vi "Store Panel by Section.vi"(8 "error in (no error)":errorcluster, 9 "Show Status? (T)":bool=TRUE, 10 "VI reference":refnum<vi>, 11 "Path (dialog)":path=path "C:/ProgramData/EPL/CFTS Defaults.ini") -> (0 "Error Out":errorcluster)   [LabVIEW 2020]
doc: "Store the values in the controls of a front panel in a file.\n\nFreeware from Moore Good Ideas, www.mooregoodideas.com. Do not remove this line.\ndavid@mooregoodideas.com"
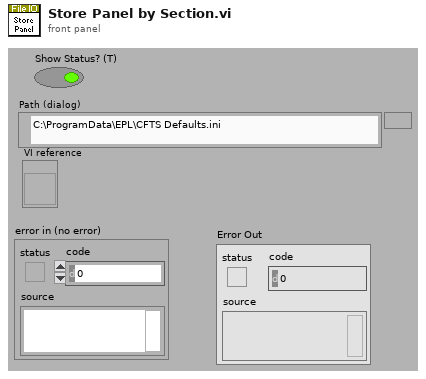
[diagram p1: front panel]
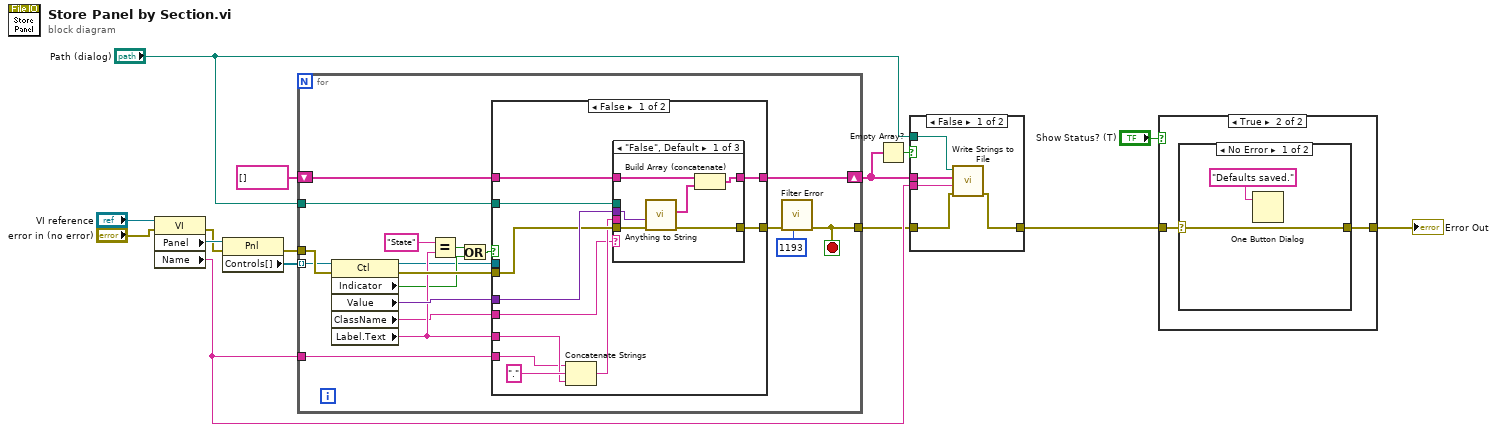
[diagram p0: block diagram]
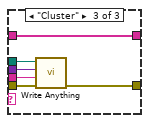
[diagram p4: hidden frame]
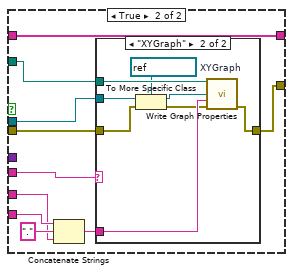
[diagram p5: hidden frame]
diagram:
  n1 = property class="VI"(reference="VI reference", error in="error in (no error)") -> (error out=w10:errorcluster, "Panel"=w11:refnum<vi>, "Name"=w4:string)  [unwired: 1 out]
  n2 = property class="Pnl"(reference=w11, error in=w10) -> (error out=w8:errorcluster, "Controls[]"=w9:refnum<vi>[])  [unwired: 1 out]
  n3 = for {
    tunnel: w9 -> [w27] mode=indexing
    tunnel: w8 -> [w33]
    tunnel: [w26] -> w2
    tunnel: "Path (dialog)" -> [w30]
    tunnel: w4 -> [w28]
    shift-right: [w24] -> w6
    shift-left: string[] [] -> [w23]
    stop <- w26 stop-if-true
    n4 = property class="Ctl"(reference=w27, error in=w33) -> (reference out=w16:refnum<vi>, error out=w31:errorcluster, "Indicator"=w19:bool, "Value"=w32:variant, "ClassName"=w17:string, "Label.Text"=w22:string)
    n5 = Equal?(x="State", y=w22) -> (x = y?=w20:bool)
    n6 = Or(x=w20, y=w19) -> (x .or. y?=w18:bool)
    n7 = case shown="False" w18 {
      tunnel: w32 -> [w44 _]
      tunnel: [w43 w60] -> w29
      tunnel: w31 -> [w41 w61]
      tunnel: w30 -> [w42 w63]
      tunnel: w28 -> [w38 w66]
      tunnel: w22 -> [w39 w65]
      tunnel: w17 -> [w34 w64]
      tunnel: [w36 w68] -> w24
      tunnel: w23 -> [w35 w68]
      tunnel: w16 -> [_ w62]
      frame False {
        n8 = Concatenate Strings(w38, "." ("string"), w39) -> (w37:string)
        n9 = case shown="\"False\", Default" w34 {
          tunnel: w44 -> [w49 _ w58]
          tunnel: [w50 w52 w57] -> w43
          tunnel: w42 -> [_ _ w56]
          tunnel: w41 -> [w48 w52 w55]
          tunnel: w37 -> [_ _ w54]
          tunnel: [w46 w51 w53] -> w36
          tunnel: w35 -> [w45 w51 w53]
          frame "False", Default {
            n10 = call "Anything to String.vi"("Error In"=w48, "Anything"=w49) -> ("Error Out"=w50:errorcluster, "Strings[]"=w47:string[])  [unwired: 7 in, 1 out]
            n11 = Build Array (concatenate)(w45, w47) -> (w46:string[])
          }
          frame "" {
          }
          frame "Cluster" {
            n12 = call "Write Anything.vi"("Error In"=w55, "Section Name (Name of \"Anything\")"=w54, "Anything"=w58, "Path (dialog)"=w56) -> ("Error Out"=w57:errorcluster)  [unwired: 7 out]
          }
        }
      }
      frame True {
        n13 = Concatenate Strings(w66, "." ("string"), w65) -> (w59:string)
        n14 = case shown="\"XYGraph\"" w64 {
          tunnel: w63 -> [_ w77]
          tunnel: w62 -> [_ w74]
          tunnel: w61 -> [w69 w73]
          tunnel: [w69 w76] -> w60
          tunnel: w59 -> [_ w75]
          frame "False", Default {
          }
          frame "XYGraph" {
            w71 = refnum<vi> refnum  # XYGraph
            n15 = To More Specific Class(target class=w71, reference=w74, error in=w73) -> (specific class reference=w70:refnum<vi>, error out=w72:errorcluster)
            n16 = call "Write Graph Properties.vi"("Config File"=w77, "WFGraph Refnum"=w70, "Section"=w75, "error in (no error)"=w72) -> ("error out"=w76:errorcluster)  [unwired: 11 in]
          }
        }
      }
    }
    n17 = call "Filter Error.vi"("error in (no error)"=w29, "code to ignore"=1193) -> ("error out"=w26:errorcluster)  [unwired: 9 in]
  }
  n18 = Empty Array?(array=w6) -> (empty?=w5:bool)
  n19 = case shown="False" w5 {
    tunnel: w6 -> [w79 _]
    tunnel: w4 -> [w78 _]
    tunnel: "Path (dialog)" -> [w82 _]
    tunnel: w2 -> [w81 w83]
    tunnel: [w80 w83] -> w1
    frame False {
      n20 = call "Write Strings to File.vi"("Error In"=w81, "Section Name"=w78, "Array of Strings"=w79, "Path"=w82) -> ("Error Out"=w80:errorcluster)  [unwired: 7 in]
    }
    frame True {
    }
  }
  n21 = case shown="True" "Show Status? (T)" {
    tunnel: w1 -> [w84 w86]
    tunnel: [w84 w85] -> w12
    frame False {
    }
    frame True {
      n22 = case shown="No Error" w86 {
        selector: w86 -> [w87 w89]
        tunnel: [w87 w89] -> w85
        frame No Error {
          n23 = One Button Dialog(message="Defaults saved.") -> ()  [unwired: 1 in, 1 out]
        }
        frame Error {
        }
      }
    }
  }
  "Error Out" <- w12
